vi "test validation.vi"() -> (0 "Error 42":errorcluster, 1 "no error":errorcluster)   [LabVIEW 2025, in "NISE_CEF_Tests.lvlib"]
uses:
  NISE_CEF_Tests.lvlib
  Trunk/Configuration Framework/serializable configuration/NISE_CEF_serializable configuration.lvclass
  Trunk/ProjectTemplates/Source/Advanced Configurator/Classes/channel configuration/channel configuration.lvclass
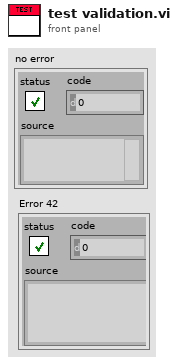
[diagram p1: front panel]
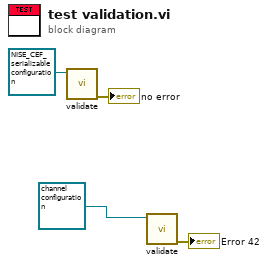
[diagram p0: block diagram]
diagram:
  n1 = call-dynamic "validate.vi"("configuration in"=refnum<class "NISE_CEF_serializable configuration.lvclass"> refnum ("configuration")) -> ("error out"=→"no error":errorcluster)  [unwired: 9 in, 1 out]
  n2 = call-dynamic "validate.vi"("configuration in"=refnum<class "channel configuration.lvclass"> refnum ("channel configuration.lvclass")) -> ("error out"=→"Error 42":errorcluster)  [unwired: 9 in, 1 out]
